vi "UHR-Fleezers Control (host) -Leonardo 04-2018 V3_greenctrl.vi"(0 "Tab Green FB":T5(tab)=enum."Trap Control (RF)") -> ()   [LabVIEW 2013] (continued)
              }
              n1852 = for {
                tunnel: w3550 -> [w3569] mode=indexing
                tunnel: [w3568] -> w3560 mode=indexing
                workers-P: _ -> [_]
                n1853 = Unbundle By Name(w3569) -> ("magnitude"=w3568:dbl[])
              }
              n1854 = Transpose 2D Array(2D array=w3560) -> (transposed array=w3559:dbl[][])
              n1855 = for {
                tunnel: w3559 -> [w3567] mode=indexing
                tunnel: [w3566] -> w3558 mode=indexing
                workers-P: _ -> [_]
                n1856 = Add Array Elements(numeric array=w3567) -> (sum=w3566:dbl)
              }
              n1857 = Select(t=w3553, s=w3554, f=w3552) -> (s? t:f=w3551:dbl)
              n1858 = Divide(x=w3558, y=w3551) -> (x/y=w3556:dbl[])
              n1859 = Bundle By Name(cluster=w3557, "magnitude"=w3556) -> (w3555:cluster{"f0":dbl, "df":dbl, "magnitude":dbl[]})
            }
          }
        }
        n1860 = case shown="True" w3497 {
          tunnel: w3498 -> [w3529 w3535]
          tunnel: [w3529 w3530] -> w3496
          frame False {
          }
          frame True {
            n1861 = Array Subset(array=w3535, index (row)=0 ("index"), length (row)=4 ("length"), index (col)=0 ("index"), length (col)=1 ("length")) -> (w3530:T47)
          }
        }
        n1862 = feedback-in #9(w3496) -> ()
        n1863 = Split 1D Array(array=w3510, index=2) -> (first subarray=→"FFT 1":cluster{"f0":dbl, "df":dbl, "magnitude":dbl[]}[], second subarray=→"FFT 2":cluster{"f0":dbl, "df":dbl, "magnitude":dbl[]}[])
      }
    }
    n1864 = Index Array(array=w2392, index=1) -> (element=w2400:waveform(dbl))
    n1865 = case "For displaying the high resolution display (no downsampling)" shown="True" w2456 {
      tunnel: w2419 -> [_ w2738]
      frame False {
      }
      frame True {
        n1866 = Index Array(array=w2738, index="High Res. Display") -> (element=w2739:waveform(dbl))
        n1867 = call <vilib>:"Std Deviation and Variance.vi"("X"=w2739) -> ("mean"=w2746:dbl, "standard deviation"=w2751:dbl)  [unwired: 1 in, 1 out]
        "Mean Intensity" <- w2746
        "Sigma" <- w2751
        n1868 = Subtract(x=w2739, y=w2746) -> (x-y=w2745:waveform(dbl))
        n1869 = Select(t=w2745, s="Subtract mean", f=w2739) -> (s? t:f=→"1 Channel":waveform(dbl))
        n1870 = Divide(x=w2751, y=w2746) -> (x/y=→"Sigma/Mean":dbl)
        n1871 = feedback #10(1) -> (w2740:i32)
        n1872 = Greater Or Equal?(x=w2740, y="Slow mean N ave.") -> (x >= y?=w2753:bool)
        n1873 = Increment(x=w2740) -> (x+1=w2755:i32)
        n1874 = Select(t=1, s=w2753, f=w2755) -> (s? t:f=w2742:i32)
        n1875 = feedback-in #10(w2742) -> ()
        n1876 = feedback #11() -> (w2743:waveform(dbl))  [unwired: 1 out]
        n1877 = case shown="Default" w2740 {
          tunnel: [w2758 w2761] -> w2744
          tunnel: w2743 -> [w2760 _]
          tunnel: w2739 -> [w2759 w2761]
          frame Default {
            n1878 = call-poly <vilib>:"Append Waveforms.vi"("waveform B"=w2759, "waveform A"=w2760) -> ("waveform out"=w2758:waveform(dbl))  [unwired: 1 in, 8 out]
          }
          frame 1 {
          }
        }
        n1879 = feedback-in #11(w2744) -> ()
        n1880 = case shown="True" w2753 {
          tunnel: w2744 -> [_ w2757]
          frame False {
          }
          frame True {
            n1881 = call-poly <vilib>:"Mean.vi"("X"=w2757) -> ("mean"=→"Slow mean":dbl)  [unwired: 1 out]
          }
        }
      }
    }
    n1882 = case "For plotting results of scanning MCL" shown="True" w2526 {
      tunnel: w2525 -> [_ w2878]
      tunnel: w2449 -> [_ w2974]
      tunnel: w2534 -> [_ _]
      tunnel: w2419 -> [_ w2948]
      tunnel: w2394 -> [_ w2879]
      tunnel: w2393 -> [_ w2852]
      frame False {
      }
      frame True {
        w2859 = u32 0 items=["Horizontal", "Vertical", "Central", "1st Diagonal", "2nd Diagonal"] ("Type of Symmetry")
        w2887 = u32 0 items=["Horizontal", "Vertical", "Central", "1st Diagonal", "2nd Diagonal"] ("Type of Symmetry")
        w2890 = u32 0 items=["Horizontal", "Vertical", "Central", "1st Diagonal", "2nd Diagonal"] ("Type of Symmetry")
        w2919 = u32 0 items=["Horizontal", "Vertical", "Central", "1st Diagonal", "2nd Diagonal"] ("Type of Symmetry")
        n1883 = Index Array(array=w2948, index=10) -> (element=w2954:waveform(dbl))
        n1884 = Index Array(array=w2948, index=11) -> (element=w2951:waveform(dbl))
        n1885 = local read "Cycles/step (MCL)"() -> (w2904:u64)
        n1886 = Index Array(array=w2948, index="Channel") -> (element=w2950:waveform(dbl))
        n1887 = Unbundle(w2852) -> ("New Image"=w2851:T3, "New Image"=w2850:T3, "New Image"=w2849:T3, "New Image"=w2848:T3)
        n1888 = Unbundle By Name(w2954) -> ("Y"=w2906:dbl[])
        n1889 = Unbundle By Name(w2951) -> ("Y"=w2908:dbl[])
        n1890 = Unbundle By Name(w2950) -> ("Y"=w2913:dbl[])
        n1891 = call "downsample 1D array - double.vi"("Ave N"=w2904, "Array In"=w2906) -> ("Array Out"=w2905:dbl[])  [unwired: 1 out]
        n1892 = call "downsample 1D array - double.vi"("Ave N"=w2904, "Array In"=w2908) -> ("Array Out"=w2907:dbl[])  [unwired: 1 out]
        n1893 = call "downsample 1D array - double.vi"("Ave N"=w2904, "Array In"=w2913) -> ("Array Out"=w2912:dbl[])  [unwired: 1 out]
        n1894 = feedback #12(w2974) -> (w2975:dbl[])
        n1895 = Build Array (concatenate)(w2975, w2974) -> (w2956:dbl[])
        n1896 = feedback #13(w2879) -> (w2881:dbl[])
        n1897 = Build Array (concatenate)(w2881, w2879) -> (w2880:dbl[])
        n1898 = local read "Scan steps (MCL)"() -> (w2861:u64)
        n1899 = Select(t=w2974, s=w2878, f=w2956) -> (s? t:f=w2960:dbl[])
        n1900 = feedback-in #12(w2960) -> ()
        n1901 = Select(t=w2879, s=w2878, f=w2880) -> (s? t:f=w2862:dbl[])
        n1902 = feedback-in #13(w2862) -> ()
        n1903 = local read "Scan lines (y)"() -> (w2847:u64)
        n1904 = local read "N APD Samp/step"() -> (w2863:dbl)
        n1905 = feedback #14(w2905) -> (w2962:dbl[])
        n1906 = Build Array (concatenate)(w2962, w2905) -> (w2953:dbl[])
        n1907 = feedback #15(w2912) -> (w2972:dbl[])
        n1908 = Build Array (concatenate)(w2972, w2912) -> (w2971:dbl[])
        n1909 = feedback #16(w2907) -> (w2964:dbl[])
        n1910 = Build Array (concatenate)(w2964, w2907) -> (w2965:dbl[])
        n1911 = Select(t=w2905, s=w2878, f=w2953) -> (s? t:f=w2909:dbl[])
        n1912 = feedback-in #14(w2909) -> ()
        n1913 = Select(t=w2912, s=w2878, f=w2971) -> (s? t:f=w2911:dbl[])
        n1914 = feedback-in #15(w2911) -> ()
        n1915 = Select(t=w2907, s=w2878, f=w2965) -> (s? t:f=w2910:dbl[])
        n1916 = feedback-in #16(w2910) -> ()
        n1917 = Multiply(x=w2861, y=u64 2) -> (x*y=w2846:u64)
        n1918 = call "integrate 1D array interval - double.vi"("Ave N"=w2863, "Array In"=w2862) -> ("Array Out"=w2874:dbl[])  [unwired: 1 out]
        n1919 = call "integrate 1D array interval - double.vi"("Ave N"=w2863, "Array In"=w2960) -> ("Array Out"=w2959:dbl[])  [unwired: 1 out]
        n1920 = Array Size(array=w2874) -> (size(s)=w2875:i32)
        n1921 = Array Size(array=w2959) -> (size(s)=w2961:i32)
        n1922 = Multiply(x=w2847, y=w2846) -> (x*y=w2877:u64)
        n1923 = Multiply(x=w2847, y=w2846) -> (x*y=w2969:u64)
        n1924 = call-poly <vilib>:"Mean.vi"("X"=w2909) -> ("mean"=w2893:dbl)  [unwired: 1 out]
        n1925 = Subtract(x=w2877, y=w2875) -> (x-y=w2868:u64)
        n1926 = call-poly <vilib>:"Mean.vi"("X"=w2911) -> ("mean"=w2898:dbl)  [unwired: 1 out]
        n1927 = call-poly <vilib>:"Mean.vi"("X"=w2910) -> ("mean"=w2896:dbl)  [unwired: 1 out]
        n1928 = call-poly <vilib>:"Mean.vi"("X"=w2874) -> ("mean"=w2865:dbl)  [unwired: 1 out]
        n1929 = Subtract(x=w2969, y=w2961) -> (x-y=w2903:u64)
        n1930 = call-poly <vilib>:"Mean.vi"("X"=w2959) -> ("mean"=w2900:dbl)  [unwired: 1 out]
        n1931 = Initialize Array(1.0 ("element"), w2868) -> (w2864:dbl[])
        n1932 = Initialize Array(1.0 ("element"), w2903) -> (w2894:dbl[])
        n1933 = Multiply(x=w2864, y=w2865) -> (x*y=w2866:dbl[])
        n1934 = Multiply(x=w2894, y=w2896) -> (x*y=w2897:dbl[])
        n1935 = Multiply(x=w2894, y=w2898) -> (x*y=w2899:dbl[])
        n1936 = Multiply(x=w2894, y=w2893) -> (x*y=w2895:dbl[])
        n1937 = Multiply(x=w2894, y=w2900) -> (x*y=w2901:dbl[])
        n1938 = Build Array (concatenate)(w2909, w2895) -> (w2963:dbl[])
        n1939 = Build Array (concatenate)(w2911, w2899) -> (w2967:dbl[])
        n1940 = Build Array (concatenate)(w2910, w2897) -> (w2966:dbl[])
        n1941 = Build Array (concatenate)(w2874, w2866) -> (w2876:dbl[])
        n1942 = Build Array (concatenate)(w2959, w2901) -> (w2968:dbl[])
        n1943 = Reshape Array(w2963, w2847, w2846) -> (w2929:dbl[][])
        n1944 = Reshape Array(w2876, w2847, w2846) -> (w2872:dbl[][])
        n1945 = Reshape Array(w2967, w2847, w2846) -> (w2921:dbl[][])
        n1946 = Reshape Array(w2966, w2847, w2846) -> (w2936:dbl[][])
        n1947 = Reshape Array(w2968, w2847, w2846) -> (w2946:dbl[][])
        n1948 = Array Subset(array=w2936, index (col)=0 ("index"), length (col)=w2861) -> (w2941:dbl[][])  [unwired: 2 in]
        n1949 = Array Subset(array=w2936, index (col)=w2861) -> (w2939:dbl[][])  [unwired: 3 in]
        n1950 = Array Subset(array=w2921, index (col)=0 ("index"), length (col)=w2861) -> (w2927:dbl[][])  [unwired: 2 in]
        n1951 = Array Subset(array=w2921, index (col)=w2861) -> (w2925:dbl[][])  [unwired: 3 in]
        n1952 = Array Subset(array=w2872, index (col)=0 ("index"), length (col)=w2861) -> (w2871:dbl[][])  [unwired: 2 in]
        n1953 = Array Subset(array=w2872, index (col)=w2861) -> (w2869:dbl[][])  [unwired: 3 in]
        n1954 = Array Subset(array=w2946, index (col)=0 ("index"), length (col)=w2861) -> (w2945:dbl[][])  [unwired: 2 in]
        n1955 = Array Subset(array=w2946, index (col)=w2861) -> (w2943:dbl[][])  [unwired: 3 in]
        n1956 = Array Subset(array=w2929, index (col)=0 ("index"), length (col)=w2861) -> (w2934:dbl[][])  [unwired: 2 in]
        n1957 = Array Subset(array=w2929, index (col)=w2861) -> (w2932:dbl[][])  [unwired: 3 in]
        n1958 = for {
          tunnel: w2941 -> [w2983] mode=indexing
          tunnel: [w2982] -> w2940 mode=indexing
          workers-P: _ -> [_]
          n1959 = Reverse 1D Array(array=w2983) -> (reversed array=w2982:dbl[])
        }
        n1960 = for {
          tunnel: w2927 -> [w2979] mode=indexing
          tunnel: [w2978] -> w2926 mode=indexing
          workers-P: _ -> [_]
          n1961 = Reverse 1D Array(array=w2979) -> (reversed array=w2978:dbl[])
        }
        n1962 = for {
          tunnel: w2871 -> [w2977] mode=indexing
          tunnel: [w2976] -> w2870 mode=indexing
          workers-P: _ -> [_]
          n1963 = Reverse 1D Array(array=w2977) -> (reversed array=w2976:dbl[])
        }
        n1964 = for {
          tunnel: w2945 -> [w2985] mode=indexing
          tunnel: [w2984] -> w2944 mode=indexing
          workers-P: _ -> [_]
          n1965 = Reverse 1D Array(array=w2985) -> (reversed array=w2984:dbl[])
        }
        n1966 = for {
          tunnel: w2934 -> [w2981] mode=indexing
          tunnel: [w2980] -> w2933 mode=indexing
          workers-P: _ -> [_]
          n1967 = Reverse 1D Array(array=w2981) -> (reversed array=w2980:dbl[])
        }
        n1968 = Index Array(array=w2946, index (row)=0) -> (element=→"Waveform Graph":dbl[])  [unwired: 1 in]
        n1969 = Add(x=w2940, y=w2939) -> (x+y=w2938:dbl[][])
        n1970 = Add(x=w2926, y=w2925) -> (x+y=w2924:dbl[][])
        n1971 = Add(x=w2870, y=w2869) -> (x+y=w2854:dbl[][])
        n1972 = Add(x=w2944, y=w2943) -> (x+y=w2918:dbl[][])
        n1973 = Add(x=w2933, y=w2932) -> (x+y=w2931:dbl[][])
        n1974 = Divide(x=w2924, y=2) -> (x/y=w2922:dbl[][])
        n1975 = Divide(x=w2938, y=2) -> (x/y=w2883:dbl[][])
        n1976 = Divide(x=w2931, y=2) -> (x/y=w2885:dbl[][])
        n1977 = To Single Precision Float(number=w2918) -> (single precision float=w2917:sgl[][])
        n1978 = Transpose 2D Array(2D array=w2922) -> (transposed array=→"Data map":dbl[][])
        n1979 = To Single Precision Float(number=w2854) -> (single precision float=w2858:sgl[][])
        n1980 = To Single Precision Float(number=w2883) -> (single precision float=w2889:sgl[][])
        n1981 = To Single Precision Float(number=w2885) -> (single precision float=w2886:sgl[][])
        n1982 = call "IMAQ ArrayToImage"("Image Pixels (Float)"=w2917, "Image"=w2851) -> ("Image Out"=w2920:T3)  [unwired: 8 in, 1 out]
        n1983 = call "IMAQ ArrayToImage"("Image Pixels (Float)"=w2858, "Image"=w2850) -> ("Image Out"=w2860:T3)  [unwired: 8 in, 1 out]
        n1984 = call "IMAQ ArrayToImage"("Image Pixels (Float)"=w2889, "Image"=w2849) -> ("Image Out"=w2891:T3)  [unwired: 8 in, 1 out]
        n1985 = call "IMAQ ArrayToImage"("Image Pixels (Float)"=w2886, "Image"=w2848) -> ("Image Out"=w2888:T3)  [unwired: 8 in, 1 out]
        n1986 = call "IMAQ Symmetry"("Type of Symmetry"=w2919, "Image Src"=w2920) -> ("Image Dst Out"=w2915:T3)  [unwired: 3 in, 1 out]
        n1987 = call "IMAQ Symmetry"("Type of Symmetry"=w2859, "Image Src"=w2860) -> ("Image Dst Out"=w2856:T3)  [unwired: 3 in, 1 out]
        n1988 = call "IMAQ Symmetry"("Type of Symmetry"=w2890, "Image Src"=w2891) -> ("Image Dst Out"=→"Detection Laser X":T3)  [unwired: 3 in, 1 out]
        n1989 = call "IMAQ Symmetry"("Type of Symmetry"=w2887, "Image Src"=w2888) -> ("Image Dst Out"=→"Detection Laser Y":T3)  [unwired: 3 in, 1 out]
        n1990 = call "IMAQ Set Simple Calibration"("Calibration Axis Info"=T37 {"Origin Pixel"={"X"=0.0, "Y"=0.0}, "Angle Relative to Horizontal (deg)"=0.0, "Axis Reference"=0}, "Grid Descriptor"=T38 {"X Step"=0.3, "Y Step"=0.3, "Unit"=enum."Undefined"}, "Image"=w2915) -> ("Calibrated Image"=→"APD 1":T3)  [unwired: 7 in, 1 out]
        n1991 = call "IMAQ Set Simple Calibration"("Calibration Axis Info"=T37 {"Origin Pixel"={"X"=0.0, "Y"=0.0}, "Angle Relative to Horizontal (deg)"=0.0, "Axis Reference"=0}, "Grid Descriptor"=T38 {"X Step"=0.3, "Y Step"=0.3, "Unit"=enum."Undefined"}, "Image"=w2856) -> ("Calibrated Image"=→"APD 2":T3)  [unwired: 7 in, 1 out]
      }
    }
    n1992 = Subtract(x=w2400, y="APD 2 Offset") -> (x-y=w2397:waveform(dbl))
    n1993 = Subtract(x=w2402, y="APD 1 Offset") -> (x-y=w2398:waveform(dbl))
    n1994 = Index Array(array=w2417, index=3) -> (element=w2476:waveform(dbl))
    n1995 = Index Array(array=w2417, index=6) -> (element=w2473:waveform(dbl))
    n1996 = Build Array(w2398, w2397) -> (→"APD Chart":waveform(dbl)[])
    n1997 = Array Size(array=w2466) -> (size(s)=w2514:i32)
    n1998 = call <vilib>:"Std Deviation and Variance.vi"("X"=w2410) -> ("standard deviation"=w2409:dbl)  [unwired: 1 in, 2 out]
    n1999 = Add Array Elements(numeric array=w2410) -> (sum=w2412:u32)
    n2000 = Add Array Elements(numeric array=w2466) -> (sum=w2524:u32)
    n2001 = call <vilib>:"Std Deviation and Variance.vi"("X"=w2466) -> ("standard deviation"=w2465:dbl)  [unwired: 1 in, 2 out]
    n2002 = Divide(x=w2409, y=w2408) -> (x/y=w2405:dbl)
    "Rate sigma (Hz) 2" <- w2405
    n2003 = Multiply(x=w2408, y=w2514) -> (x*y=w2411:dbl)
    "Int. Time (s)" <- w2411
    n2004 = Divide(x=w2412, y=w2411) -> (x/y=w2406:dbl)
    "APD 2 Rate (Hz)" <- w2406
    n2005 = Divide(x=w2524, y=w2411) -> (x/y=w2463:dbl)
    "APD 1 Rate (Hz)" <- w2463
    n2006 = Divide(x=w2465, y=w2408) -> (x/y=w2464:dbl)
    "Rate sigma (Hz)" <- w2464
    n2007 = Divide(x=w2405, y=w2406) -> (x/y=→"Sigma/Mean 2":dbl)
    n2008 = Divide(x=w2464, y=w2463) -> (x/y=→"Sigma/Mean":dbl)
    n2009 = case shown="2" "Calibration" {
      tunnel: "T1 alpha_x (nm/V)" -> [_ w2814 w2835]
      tunnel: "T1 kappa_x (pN/nm)" -> [_ _ w2825]
      tunnel: "T2 alpha_x (nm/V)" -> [_ w2813 w2833]
      tunnel: "T2 kappa_x (pN/nm)" -> [_ _ w2826]
      tunnel: w2476 -> [w2796 w2811 w2831]
      tunnel: w2473 -> [w2795 w2809 w2829]
      tunnel: [w2796 w2808 w2828] -> w2266
      tunnel: [w2795 w2807 w2827] -> w2272
      tunnel: ["T1 X (V)" ("Label.Text") "T1 X (nm)" ("Label.Text") "T1 X (pN)" ("Label.Text")] -> w2494
      tunnel: ["T2 X (V)" ("Label.Text") "T2 X (nm)" ("Label.Text") "T2 X (pN)" ("Label.Text")] -> w2493
      tunnel: ["Position (V)" ("Label.Text") "Position (nm)" ("Label.Text") "Force (pN)" ("Label.Text")] -> w2495
      tunnel: w2475 -> [_ w2799 w2818]
      tunnel: w2477 -> [_ w2802 w2820]
      tunnel: ["Mean (V)" ("Label.Text") "Mean (nm)" ("Label.Text") "Mean (pN)" ("Label.Text")] -> w2490
      tunnel: ["Difference (V)" ("Label.Text") "Difference (nm)" ("Label.Text") "Difference (pN)" ("Label.Text")] -> w2425
      frame 0, Default {
      }
      frame 1 {
        # "position"
        n2010 = Unbundle By Name(w2811) -> ("Y"=w2815:dbl[])
        n2011 = Unbundle By Name(w2809) -> ("Y"=w2800:dbl[])
        n2012 = Subtract(x=w2815, y=w2802) -> (x-y=w2803:dbl[])
        n2013 = Subtract(x=w2800, y=w2799) -> (x-y=w2801:dbl[])
        n2014 = Multiply(x=w2801, y=w2813) -> (x*y=w2810:dbl[])
        n2015 = Multiply(x=w2814, y=w2803) -> (x*y=w2812:dbl[])
        n2016 = Bundle By Name(cluster=w2809, "Y"=w2810) -> (w2807:waveform(dbl))
        n2017 = Bundle By Name(cluster=w2811, "Y"=w2812) -> (w2808:waveform(dbl))
      }
      frame 2 {
        # "force"
        n2018 = Unbundle By Name(w2831) -> ("Y"=w2836:dbl[])
        n2019 = Unbundle By Name(w2829) -> ("Y"=w2834:dbl[])
        n2020 = Subtract(x=w2834, y=w2818) -> (x-y=w2819:dbl[])
        n2021 = Subtract(x=w2836, y=w2820) -> (x-y=w2821:dbl[])
        n2022 = Compound Arithmetic op=MULTIPLY(w2819, w2833, w2826) -> (w2830:dbl[])
        n2023 = Compound Arithmetic op=MULTIPLY(w2825, w2835, w2821) -> (w2832:dbl[])
        n2024 = Bundle By Name(cluster=w2829, "Y"=w2830) -> (w2827:waveform(dbl))
        n2025 = Bundle By Name(cluster=w2831, "Y"=w2832) -> (w2828:waveform(dbl))
      }
    }
    n2026 = feedback-in #17("Calibration") -> ()
    n2027 = feedback #17(u16 1 ("Calibration")) -> (w2497:u16)
    n2028 = local read "Trap 2 Bead Size (nm)"() -> (w2305:dbl)
    n2029 = local read "Trap 1 Bead Size (nm)"() -> (w2304:dbl)
    n2030 = local read "AOM X Cal (nm/MHz)"() -> (w2302:dbl)
    n2031 = local read "Trap Delta (MHz)"() -> (w2301:dbl)
    n2032 = Not Equal?(x=w2497, y="Calibration") -> (x != y?=w2454:bool)
    n2033 = Multiply(x=w2302, y=w2301) -> (x*y=w2306:dbl)
    n2034 = Unbundle By Name(w2266) -> ("Y"=w2271:dbl[])
    n2035 = Unbundle By Name(w2272) -> ("Y"=w2270:dbl[])
    n2036 = Add(x=w2305, y=w2304) -> (x+y=w2308:dbl)
    n2037 = case shown="False" "Negate trap 2 force" {
      tunnel: [-1.0 1.0] -> w2483
      frame False {
      }
      frame True {
      }
    }
    n2038 = Unbundle By Name(w2476) -> ("Y"=w2479:dbl[])
    n2039 = Unbundle By Name(w2473) -> ("Y"=w2482:dbl[])
    n2040 = Divide(x=w2308, y=2.0) -> (x/y=w2303:dbl)
    n2041 = Subtract(x=w2271, y=w2270) -> (x-y=w2268:dbl[])
    n2042 = Subtract(x=w2479, y=w2477) -> (x-y=w2480:dbl[])
    n2043 = Subtract(x=w2482, y=w2475) -> (x-y=w2481:dbl[])
    n2044 = Divide(x=w2268, y=2.0) -> (x/y=w2267:dbl[])
    n2045 = Multiply(x=w2481, y="T2 alpha_x (nm/V)") -> (x*y=w2472:dbl[])
    n2046 = Multiply(x="T1 alpha_x (nm/V)", y=w2480) -> (x*y=w2471:dbl[])
    n2047 = Multiply(x=w2272, y=w2483) -> (x*y=w2484:waveform(dbl))
    n2048 = Bundle By Name(cluster=w2266, "Y"=w2267) -> (w2265:waveform(dbl))
    n2049 = case shown="True" "Read Lateness and Rel Phase" {
      tunnel: w2278 -> [w2762 w2784]
      tunnel: w2317 -> [w2763 w2783]
      tunnel: [w2762 w2782] -> w2469
      tunnel: [w2763 w2781] -> w2468
      frame False {
      }
      frame True {
        n2050 = xnode "Read/Write Control"("FPGA VI Reference In"=w2784, "error in"=w2783) -> ("FPGA VI Reference Out"=w2782:T20, "error out"=w2781:errorcluster, "GI Relative phase"=→"GI relative phase":i16, "Relative phase"=→"Relative phase (AI1)":i16, "AI Late Counter"=→"Late Counter (AI1)":u8, "GI Late Counter"=→"GI Late Counter":u8, "MCL Late Counter"=→"MCL Late Counter":u8, "MCL Relative Phase"=→"Relative Phase (MCL)":i16, "APD Acq Relative Phase"=→"APD Acq Relative Phase":i16, "APD 1 Gate Relative Phase"=→"APD 1 Gate Relative Phase":i16, "APD 2 Gate Relative Phase"=→"APD 2 Gate Relative Phase":i16, "APD Acq Late Counter"=→"APD Acq Late Counter":u16, "APD 1 Gate Late Counter"=→"APD 1 Gate Late Counter":u8, "APD 2 Gate Late Counter"=→"APD 2 Gate Late Counter":u8, "Green FB Relative Phase"=→"Relative phase (Green FB)":i16, "GI Relative phase"=→"GI relative phase 2":i16, "GI Late Counter 2"=→"GI Late Counter 2":u16, "Trap Pos FIFO Timeout"=→"Trap Pos FIFO Timeout":u16, "Trap AI FIFO Timeout"=→"Trap AI FIFO Timeout":u16)
      }
    }
    n2051 = Subtract(x=w2472, y=w2471) -> (x-y=w2300:dbl[])
    n2052 = call-poly <vilib>:"Mean.vi"("X"=w2300) -> ("mean"=w2307:dbl)  [unwired: 1 out]
    n2053 = Add(x=w2306, y=w2307) -> (x+y=w2310:dbl)
    n2054 = Subtract(x=w2310, y=w2303) -> (x-y=→"Tether Extension (nm, calculated)":dbl)
    n2055 = Unbundle By Name(w2272) -> ("Y"=w2263:dbl[])
    n2056 = Unbundle By Name(w2266) -> ("Y"=w2264:dbl[])
    n2057 = Build Array(w2266, w2484, w2265) -> (→"Force":waveform(dbl)[])
    n2058 = Subtract(x=w2300, y="Offset (nm)") -> (x-y=w2444:dbl[])
    n2059 = call-poly <vilib>:"Mean.vi"("X"=w2263) -> ("mean"=w2261:dbl)  [unwired: 1 out]
    "T2 X" <- w2261
    n2060 = call-poly <vilib>:"Mean.vi"("X"=w2264) -> ("mean"=w2262:dbl)  [unwired: 1 out]
    "T1 X" <- w2262
    n2061 = Subtract(x=w2264, y=w2263) -> (x-y=w2446:dbl[])
    n2062 = Bundle By Name(cluster=w2476, "Y"=w2444) -> (w2416:waveform(dbl))
    "Bead Separation" <- w2416
    n2063 = Divide(x=w2446, y=2.0) -> (x/y=→"Vec Mean of T1 T2":dbl[])
    n2064 = case shown="True" w2454 {
      tunnel: w2495 -> [_ w2789]
      tunnel: w2494 -> [_ w2788]
      tunnel: w2493 -> [_ w2787]
      tunnel: w2490 -> [_ w2786]
      tunnel: w2425 -> [_ w2785]
      frame False {
      }
      frame True {
        n2065 = property on="Force" class="WFChart (strict)"("YScale.NameLbl.Text"=w2789) -> ()  [unwired: 2 in, 2 out]
        n2066 = property on="T2 X" class="DigNum (strict)"("Caption.Text"=w2787) -> ()  [unwired: 2 in, 2 out]
        n2067 = property on="T1 X" class="DigNum (strict)"("Caption.Text"=w2788) -> ()  [unwired: 2 in, 2 out]
        n2068 = property on="Mean" class="DigNum (strict)"("Caption.Text"=w2786) -> ()  [unwired: 2 in, 2 out]
        n2069 = property on="Difference" class="DigNum (strict)"("Caption.Text"=w2785) -> ()  [unwired: 2 in, 2 out]
      }
    }
    n2070 = local read "Tether"() -> (w2448:bool)
    n2071 = Subtract(x=w2262, y=w2261) -> (x-y=w2492:dbl)
    n2072 = Add(x=w2262, y=w2261) -> (x+y=→"Difference":dbl)
    n2073 = feedback #18(w2444) -> (w2443:dbl[])
    n2074 = Divide(x=w2492, y=2.0) -> (x/y=w2275:dbl)
    "Mean" <- w2275
    n2075 = case shown="True" w2448 {
      tunnel: w2275 -> [_ w2721]
      frame False {
      }
      frame True {
        n2076 = Greater?(x="Lost Tether Alarm Threshold (pN)", y=w2721) -> (0:w2719:bool)
        n2077 = case shown="True" w2719 {
          frame False {
          }
          frame True {
            n2078 = flat-sequence {
              frame #0 {
                # "stop only if saving"
                n2079 = local read "Saving..."() -> (w2734:bool)
                n2080 = And(x=w2734, y="TA Cancel Save?") -> (x .and. y?=w2733:bool)
                n2081 = local write "Stop Saving"(w2733) -> ()
              }
              frame #1 {
                n2082 = case shown="True" "TA Green Off?" {
                  frame False {
                  }
                  frame True {
                    w2737 = FALSE ("Fl. Triggered...")
                    n2083 = local write "Fl. Triggered..."(w2737) -> ()
                    n2084 = property on="Green Laser ON/Interlacing" class="Bool (strict)"("Val(Sgnl)"=w2737) -> ()  [unwired: 2 in, 2 out]
                  }
                }
              }
            }
            n2085 = local read "Time tether formed"() -> (w2728:timestamp)
            n2086 = Get Date/Time In Seconds() -> (seconds since 1Jan1904=w2729:timestamp)
            n2087 = Subtract(x=w2729, y=w2728) -> (x-y=w2727:dbl)
            n2088 = Number To Decimal String(number=w2727) -> (decimal integer string=w2724:string)  [unwired: 1 out]
            n2089 = local read "Messages"() -> (w2731:string)
            n2090 = call <vilib>:"Beep.vi"() -> ()  [unwired: 3 in, 9 out]
            n2091 = Concatenate Strings("Lost tether (" ("Message to add"), w2724, " s)." ("string")) -> (w2726:string)
            n2092 = local write "Tether"(FALSE ("Tether")) -> ()
            n2093 = call "Update messages.vi"("Message to add"=w2726, "Old message string"=w2731) -> ("New message string"=w2730:string)
            n2094 = local write "Messages"(w2730) -> ()
            n2095 = property on="Trap Pos. FB ON" class="Bool (strict)"("Val(Sgnl)"=FALSE ("Value (Signaling)")) -> ()  [unwired: 2 in, 2 out]
          }
        }
      }
    }
    n2096 = Build Array (concatenate)(w2444, w2443) -> (w2442:dbl[])
    n2097 = Split 1D Array(array=w2442, index=w2328) -> (first subarray=w2438:dbl[])  [unwired: 1 out]
    n2098 = feedback-in #18(w2438) -> ()
    n2099 = call-poly <vilib>:"Mean.vi"("X"=w2438) -> ("mean"=w2437:dbl)  [unwired: 1 out]
    "Bead Mean (nm)" <- w2437
    n2100 = Subtract(x=w2438, y=w2437) -> (x-y=w2436:dbl[])
    n2101 = Square(x=w2436) -> (x^2=w2435:dbl[])
    n2102 = case shown="True" "Semi Passive ON" {
      tunnel: "Semi Passive mode" -> [_ w2602]
      tunnel: "Jump Force (pN)" -> [_ w2601]
      tunnel: w2275 -> [_ w2600]
      frame False {
      }
      frame True {
        n2103 = case shown="\"Use Feedback\"" w2602 {
          tunnel: w2601 -> [_ w2605 w2621]
          tunnel: w2600 -> [_ w2604 w2620]
          frame "None" {
          }
          frame "Use Feedback" {
            n2104 = local read "Target Force (pN)"() -> (w2607:dbl)
            n2105 = Less?(x=w2605, y=w2607) -> (x < y?=w2606:bool)
            n2106 = case shown="True" w2606 {
              tunnel: w2605 -> [w2614 w2617]
              tunnel: w2604 -> [w2613 w2616]
              tunnel: [w2612 w2615] -> w2603
              frame False {
                n2107 = Less?(x=w2614, y=w2613) -> (x < y?=w2612:bool)
              }
              frame True {
                n2108 = Greater?(x=w2617, y=w2616) -> (0:w2615:bool)
              }
            }
            n2109 = case shown="True" w2603 {
              frame False {
                n2110 = local read "Trap Pos. FB ON"() -> (w2608:bool)
                n2111 = case shown="True" w2608 {
                  frame False {
                  }
                  frame True {
                    n2112 = property on="Trap Pos. FB ON" class="Bool (strict)"("Val(Sgnl)"=FALSE) -> ()  [unwired: 2 in, 2 out]
                  }
                }
              }
              frame True {
                n2113 = local read "Trap Pos. FB ON"() -> (w2610:bool)
                n2114 = case shown="False" w2610 {
                  frame False {
                    n2115 = property on="Trap Pos. FB ON" class="Bool (strict)"("Val(Sgnl)"=TRUE) -> ()  [unwired: 2 in, 2 out]
                  }
                  frame True {
                  }
                }
              }
            }
          }
          frame "Sharp Jump" {
            n2116 = local read "Target Force (pN)"() -> (w2623:dbl)
            n2117 = Greater?(x=w2621, y=w2623) -> (0:w2622:bool)
            n2118 = case shown="True" w2622 {
              tunnel: w2621 -> [w2638 w2642]
              tunnel: w2620 -> [w2639 w2641]
              tunnel: [w2637 w2640] -> w2619
              frame False {
                n2119 = Greater?(x=w2639, y=w2638) -> (0:w2637:bool)
              }
              frame True {
                n2120 = Less?(x=w2642, y=w2641) -> (x < y?=w2640:bool)
              }
            }
            n2121 = Subtract(x=w2621, y=w2623) -> (x-y=w2618:dbl)
            n2122 = case shown="True" w2619 {
              tunnel: w2618 -> [_ w2629]
              frame False {
              }
              frame True {
                n2123 = local read "T1 kappa_x (pN/nm)"() -> (w2634:dbl)
                n2124 = local read "T2 kappa_x (pN/nm)"() -> (w2635:dbl)
                n2125 = Reciprocal(x="DNA stiffness (pN / nm)") -> (1/x=w2631:dbl)
                n2126 = Reciprocal(x=w2634) -> (1/x=w2633:dbl)
                n2127 = Reciprocal(x=w2635) -> (1/x=w2632:dbl)
                n2128 = Compound Arithmetic op=ADD(w2633, w2632, w2631) -> (w2630:dbl)
                n2129 = local read "AOM X Cal (nm/MHz)"() -> (w2628:dbl)
                n2130 = Multiply(x=w2630, y=w2629) -> (x*y=w2627:dbl)
                n2131 = local read "Trap Delta (MHz)"() -> (w2625:dbl)
                n2132 = Divide(x=w2627, y=w2628) -> (x/y=w2626:dbl)
                n2133 = Subtract(x=w2625, y=w2626) -> (x-y=w2624:dbl)
                n2134 = property on="Trap Delta (MHz)" class="DigNum (strict)"("Val(Sgnl)"=w2624) -> ()  [unwired: 2 in, 2 out]
              }
            }
          }
        }
      }
    }
    n2135 = call-poly <vilib>:"Mean.vi"("X"=w2435) -> ("mean"=w2434:dbl)  [unwired: 1 out]
    n2136 = Square Root(x=w2434) -> (sqrt(x)=w2433:dbl)
    n2137 = Multiply(x=10.0, y=w2433) -> (x*y=→"RMS (Ang)":dbl)
    n2138 = xnode "Read/Write Control"("FPGA VI Reference In"=w2469, "error in"=w2468) -> ("FPGA VI Reference Out"=w2578:T20, "error out"=w2572:errorcluster, "AI2 Y Sum Set 1"=w2568:i16, "AI2 Y Sum Set 2"=w2567:i16, "AI1 X Set 1"=w2362:fxp<+/-,16,1>, "AI1 X Set 2"=w2361:fxp<+/-,16,1>, "Trap Pos FB Int Signal"=→"Trap Pos FB Int Signal":fxp<+/-,24,9>, "Trap Pos FB Int-Norm Signal"=→"Trap Pos FB Int-Norm Signal":fxp<+/-,16,1>, "Trap Pos FB Action"=w2355:i64, "Scanning"=→"AOD Scanning":bool, "Scan I"=→"AOD Scan I":u64, "Scanning MCL"=w2570:bool, "Scan I (MCL)"=→"MCL Scan I":u64, "Green FB Signals"=w2509:T48, "BD1 amplitude 1 out"=w2260:u16, "BD1 amplitude 2 out"=w2245:u16)  [unwired: 1 out]
    "MCL Scanning" <- w2570
    "Trap Pos FB Action" <- w2355
    n2139 = local read "AI2 (V)"() -> (w2569:cluster{"Set 1":dbl, "Set 2":dbl})
    n2140 = Bundle By Name(cluster=w2569, "Set 1"=w2568, "Set 2"=w2567) -> (w2565:cluster{"Set 1":dbl, "Set 2":dbl})
    n2141 = Divide(x=w2355, y=327.67) -> (x/y=→"Action (%)":dbl)
    n2142 = local read "Trap X (AI1)"() -> (w2375:T1)
    n2143 = Divide(x=w2565, y=3276.7) -> (x/y=w2564:cluster{"Set 1":dbl, "Set 2":dbl})
    n2144 = local write "AI2 (V)"(w2564) -> ()
    n2145 = Bundle(cluster=w2375, "Trap 1"=w2362, "Trap 2"=w2361) -> (→"Trap X (AI1)":T1)
    n2146 = Scale By Power Of 2(n=i16 12, x=ext 1.0) -> (x*2^n=w2256:ext)
    n2147 = Subtract(x=w2256, y=ext 1.0) -> (x-y=w2253:ext)
    n2148 = Divide(x=w2509, y=3276.7) -> (x/y=w2505:T49)
    n2149 = Multiply(x=w2260, y=ext 100.0) -> (x*y=w2254:ext)
    n2150 = Unbundle By Name(w2505) -> ("Green FB Ch 0"=w2508:dbl, "Green FB Ch 1"=w2507:dbl, "Green FB Ch 2"=w2506:dbl)
    n2151 = local read "All FB On/Off"() -> (w2244:bool)
    n2152 = Divide(x=w2254, y=w2253) -> (x/y=w2243:ext)
    "Trap 1 amplitude" <- w2243
    n2153 = Scale By Power Of 2(n=i16 12, x=ext 1.0) -> (x*2^n=w2249:ext)
    n2154 = Subtract(x=w2249, y=ext 1.0) -> (x-y=w2252:ext)
    n2155 = Multiply(x=w2245, y=ext 100.0) -> (x*y=w2251:ext)
    n2156 = Divide(x=w2508, y=w2506) -> (x/y=w2504:dbl)
    n2157 = Divide(x=w2507, y=w2506) -> (x/y=w2503:dbl)
    n2158 = flat-sequence "To save data" {
      tunnel: [w3618] -> w2589
      tunnel: [w3619] -> w2588
      tunnel: w2540 -> [w3612]
      tunnel: w2440 -> [w3616]
      tunnel: ["Save Calibration"] -> w2561
      tunnel: w2558 -> [w3615]
      tunnel: [w3608] -> w2557
      tunnel: [w3605] -> w2556
      tunnel: [w3602] -> w2555
      tunnel: w2539 -> [w3604]
      tunnel: w2452 -> [w3598]
      tunnel: [w3598] -> w2451
      tunnel: ["Start Saving"] -> w2418
      tunnel: [w3592] -> w2344
      tunnel: [w3591] -> w2343
      tunnel: w2589 -> [w3853]
      tunnel: w2588 -> [w3852]
      tunnel: w2345 -> [w3851]
      tunnel: w2561 -> [w3850]
      tunnel: w2557 -> [w3848]
      tunnel: w2556 -> [w3847]
      tunnel: w2555 -> [w3846]
      tunnel: w2427 -> [w3845]
      tunnel: w2461 -> [w3844]
      tunnel: w2451 -> [w3843]
      tunnel: w2418 -> [w3842]
      tunnel: w2416 -> [w3841]
      tunnel: w2392 -> [w3840]
      tunnel: w2344 -> [w3839]
      tunnel: w2343 -> [w3838]
      tunnel: w2342 -> [w3837]
      frame #0 {
        n2159 = Or(x="Save N Sets", y="Start Saving") -> (x .or. y?=w3599:bool)
        n2160 = To Double Precision Float(number=w3615) -> (double precision float=w3609:dbl)
        n2161 = Build Array(w3599, "Save Calibration", w3612, w3604) -> (w3614:bool[])
        n2162 = Compound Arithmetic op=OR("Save Calibration", w3612, w3599, w3604) -> (w3617:bool)
        n2163 = Boolean Array To Number(Boolean array=w3614) -> (number=w3611:u32)
        n2164 = feedback #19(FALSE ("Save APD Data\nwith Trap Data")) -> (w3593:bool)
        n2165 = feedback #20(refnum<k0> refnum) -> (w3620:refnum<file>)
        n2166 = feedback #21(refnum<k0> refnum) -> (w3595:refnum<file>)
        n2167 = feedback #22(FALSE ("Save APD Data\nwith Trap Data")) -> (w3603:bool)
        n2168 = feedback #23(refnum<k0> refnum) -> (w3606:refnum<file>)
        n2169 = feedback #24(0) -> (w3622:i32)
        n2170 = feedback #25() -> (w3610:u32)  [unwired: 1 out]
        n2171 = case shown="True" w3617 {
          tunnel: [w3629 1] -> w3618
          tunnel: w3622 -> [w3631 _]
          tunnel: [w3630 w3649] -> w3619
          tunnel: w3620 -> [w3630 _]
          tunnel: w3616 -> [_ w3669]
          tunnel: w3609 -> [_ w3667]
          tunnel: w3611 -> [_ w3670]
          tunnel: [w3628 w3648] -> w3608
          tunnel: w3610 -> [w3628 _]
          tunnel: [w3627 w3646] -> w3605
          tunnel: w3606 -> [w3627 _]
          tunnel: [w3626 w3645] -> w3602
          tunnel: w3603 -> [w3626 _]
          tunnel: "Start Saving" -> [_ w3643]
          tunnel: w3598 -> [_ w3642]
          tunnel: [w3625 w3633] -> w3591
          tunnel: w3595 -> [w3625 _]
          tunnel: [w3624 w3632] -> w3592
          tunnel: w3593 -> [w3624 _]
          frame False {
            n2172 = Increment(x=w3631) -> (x+1=w3629:i32)
          }
          frame True {
            w3639 = FALSE ("Start Saving")
            w3644 = 9.0  # File Version
            w3652 = FALSE ("prepend array or string size? (T)")
            w3650 = T30."big-endian, network order" ("byte order (0:big-endian, network order)")
            # "write file headers"
            n2173 = local read "BD 1 Frequency 1 (MHz)"() -> (w3666:dbl)
            n2174 = local read "BD 2 Frequency 1 (MHz)"() -> (w3665:dbl)
            n2175 = local read "BD 1 Frequency 2 (MHz)"() -> (w3664:dbl)
            n2176 = local read "BD 2 Frequency 2 (MHz)"() -> (w3663:dbl)
            n2177 = local read "BD 1 Frequency 3 (MHz)"() -> (w3662:dbl)
            n2178 = local read "BD 2 Frequency 3 (MHz)"() -> (w3661:dbl)
            n2179 = Array Size(array=w3642) -> (size(s)=w3641:i32)
            n2180 = To Double Precision Float(number=w3641) -> (double precision float=w3640:dbl)
            n2181 = local write "Save Calibration"(w3639) -> ()
            n2182 = local write "Start Saving"(w3639) -> ()
            n2183 = Build Array("Save APD Data\nwith Trap Data", "Save Trap Pos. Data") -> (w3636:bool[])
            n2184 = Boolean Array To Number(Boolean array=w3636) -> (number=w3635:u32)
            n2185 = Build Array(w3666, w3665, w3664, w3663, w3662, w3661) -> (w3660:dbl[])
            n2186 = case shown="2" w3670 {
              tunnel: w3669 -> [w3741 w3761 w3777 w3815]
              tunnel: w3640 -> [w3746 w3768 w3797 w3834]
              tunnel: w3667 -> [w3745 w3767 w3796 w3833]
              tunnel: [w3742 w3763 w3788 w3825] -> w3658
              tunnel: [w3733 "Cal sets to save" w3778 w3816] -> w3648
              tunnel: w3660 -> [w3743 w3764 w3790 w3827]
              tunnel: "Save APD Data\nwith Trap Data" -> [w3740 _ w3774 w3813]
              tunnel: [w3740 w3755 w3774 w3813] -> w3645
              tunnel: w3644 -> [w3736 w3756 w3772 w3811]
              tunnel: w3643 -> [w3735 _ _ _]
              tunnel: [w3726 w3755 w3771 w3801] -> w3632
              tunnel: "Save Trap Pos. Data" -> [w3726 _ w3771 w3801]
              tunnel: w3635 -> [w3725 _ w3770 w3800]
              frame 1, Default {
                # "timeseries"
                n2187 = case shown="True" "Profile" {
                  tunnel: [w3749 w3752] -> w3730
                  tunnel: [w3749 w3751] -> w3729
                  tunnel: [w3749 w3750] -> w3728
                  tunnel: [w3749 w3754] -> w3727
                  frame False {
                    w3749 = 0.0 ("f")
                  }
                  frame True {
                    n2188 = local read "Current Position"() -> (w3753:dbl[])
                    n2189 = local read "Y change (mm)"() -> (w3754:dbl)
                    n2190 = call "subVI_explode3array.vi"("Array"=w3753) -> ("x"=w3752:dbl, "y"=w3751:dbl, "z"=w3750:dbl)  [unwired: 12 in]
                  }
                }
                n2191 = local read "Save ave N"() -> (w3748:dbl)
                n2192 = Multiply(x=w3748, y=w3741) -> (x*y=w3747:dbl)
                n2193 = To Double Precision Float(number=w3725) -> (double precision float=w3739:dbl)
                n2194 = Build Array(w3736, w3741, w3747, w3746, w3745, 0.0 ("f")) -> (w3744:dbl[])
                n2195 = Build Array(w3739, w3730, w3729, w3728, w3727) -> (w3737:dbl[])
                n2196 = Select(t=u32 4000000000, s=w3735, f="N sets to save") -> (s? t:f=w3733:u32)
                n2197 = Build Array (concatenate)(w3744, w3743, w3737) -> (w3742:dbl[])
              }
              frame 2 {
                w3758 = 0.0 ("f")
                w3755 = FALSE ("Save APD Data\nwith Trap Data")
                # "calibration"
                n2198 = Boolean To (0,1)(Boolean=w3755) -> (0, 1=w3760:i16)
                n2199 = To Double Precision Float(number=w3760) -> (double precision float=w3759:dbl)
                n2200 = Build Array(w3759, w3758, w3758, w3758, w3758) -> (w3757:dbl[])
                n2201 = Build Array(w3756, w3761, w3761, w3768, w3767, 1.0 ("t")) -> (w3765:dbl[])
                n2202 = Build Array (concatenate)(w3765, w3764, w3757) -> (w3763:dbl[])
                "Calibrating Trap..." <- TRUE ("Calibrating...")
              }
              frame 4 {
                w3775 = 0.0 ("f")
                # "write file header for a trap \nraster scan"
                # "scan dir (x/y = 0/1)"
                # "cycles/step"
                # "n scans (f/b)"
                # "steps"
                # "freq. range"
                # "AOD raster scan"
                n2203 = local read "Number of F/B Scans (AOD)"() -> (w3782:u16)
                n2204 = local read "Cycles/step (AOD)"() -> (w3784:u64)
                n2205 = local read "Scan Range (MHz)"() -> (w3787:dbl)
                n2206 = local read "Scan steps (AOD)"() -> (w3786:u64)
                n2207 = local read "Scan BD"() -> (w3794:bool)
                n2208 = local read "Save ave N"() -> (w3799:dbl)
                n2209 = Boolean To (0,1)(Boolean=w3794) -> (0, 1=w3793:i16)
                n2210 = To Double Precision Float(number=w3782) -> (double precision float=w3781:dbl)
                n2211 = To Double Precision Float(number=w3786) -> (double precision float=w3785:dbl)
                n2212 = To Double Precision Float(number=w3784) -> (double precision float=w3783:dbl)
                n2213 = To Double Precision Float(number=w3793) -> (double precision float=w3792:dbl)
                n2214 = Multiply(x=w3799, y=w3777) -> (x*y=w3798:dbl)
                n2215 = To Double Precision Float(number=w3770) -> (double precision float=w3776:dbl)
                n2216 = Build Array(w3776, w3775, w3775, w3775, w3775) -> (w3773:dbl[])
                n2217 = local read "N sets should be saved"() -> (w3779:dbl)
                n2218 = Build Array(w3792, w3787, w3785, w3783, w3781) -> (w3789:dbl[])
                n2219 = Build Array(w3772, w3777, w3798, w3797, w3796, 2.0 ("t")) -> (w3791:dbl[])
                n2220 = Round Toward +Infinity(x=w3779) -> (ceil(x): smallest int >= x=w3780:dbl)
                n2221 = Build Array (concatenate)(w3791, w3790, w3773, w3789) -> (w3788:dbl[])
                n2222 = To Unsigned Long Integer(number=w3780) -> (unsigned 32bit integer=w3778:u32)
              }
              frame 8 {
                w3808 = 0.0 ("f")
                # "MCL raster scan"
                n2223 = local read "Number of scans (MCL)"() -> (w3803:u64)
                n2224 = local read "Scan lines (y)"() -> (w3802:u64)
                n2225 = local read "2D or 1D Scan"() -> (w3805:bool)
                n2226 = local read "Scan Range (V)\n(of steps)"() -> (w3824:dbl)
                n2227 = local read "Fast Scan Dir"() -> (w3831:bool)
                n2228 = local read "Cycles/step (MCL)"() -> (w3821:u64)
                n2229 = local read "Scan steps (MCL)"() -> (w3823:u64)
                n2230 = Select(t=w3802, s=w3805, f=w3803) -> (s? t:f=w3804:u64)
                n2231 = Boolean To (0,1)(Boolean=w3805) -> (0, 1=w3807:i16)
                n2232 = local read "Save ave N"() -> (w3836:dbl)
                n2233 = local read "Initial X"() -> (w3810:dbl)
                n2234 = local read "Initial Y"() -> (w3809:dbl)
                n2235 = To Double Precision Float(number=w3807) -> (double precision float=w3806:dbl)
                n2236 = Boolean To (0,1)(Boolean=w3831) -> (0, 1=w3830:i16)
                n2237 = To Double Precision Float(number=w3804) -> (double precision float=w3819:dbl)
                n2238 = To Double Precision Float(number=w3823) -> (double precision float=w3822:dbl)
                n2239 = To Double Precision Float(number=w3821) -> (double precision float=w3820:dbl)
                n2240 = To Double Precision Float(number=w3830) -> (double precision float=w3829:dbl)
                n2241 = Multiply(x=w3836, y=w3815) -> (x*y=w3835:dbl)
                n2242 = To Double Precision Float(number=w3800) -> (double precision float=w3814:dbl)
                n2243 = local read "N sets should be saved (MCL)"() -> (w3817:dbl)
                n2244 = Build Array(w3814, w3806, w3808, w3808, w3808) -> (w3812:dbl[])
                n2245 = Build Array(w3829, w3824, w3822, w3820, w3819, w3810, w3809) -> (w3826:dbl[])
                n2246 = Build Array(w3811, w3815, w3835, w3834, w3833, 3.0 ("t")) -> (w3828:dbl[])
                n2247 = Round Toward +Infinity(x=w3817) -> (ceil(x): smallest int >= x=w3818:dbl)
                n2248 = Build Array (concatenate)(w3828, w3827, w3812, w3826) -> (w3825:dbl[])
                n2249 = To Unsigned Long Integer(number=w3818) -> (unsigned 32bit integer=w3816:u32)
              }
            }
            n2250 = local read "Index"() -> (w3675:dbl)
            n2251 = call "Create new save file.vi"("Insert"="", "Ext"=".dat", "Index In"=w3675) -> ("Path Out"=w3634:path, "Index Out"=w3647:dbl)
            n2252 = local write "Save file name"(w3634) -> ()
            n2253 = local write "Index"(w3647) -> ()
            n2254 = local write "Save index"(w3647) -> ()
            n2255 = Array Size(array=w3658) -> (size(s)=w3659:i32)
            n2256 = Open/Create/Replace File(file path (use dialog)=w3634, operation (0:open)=T24."create", access (0:read/write)=enum16{"read/write", "read-only", "write-only"}."write-only") -> (refnum out=w3672:refnum<file>)  [unwired: 1 in, 4 out]
            n2257 = local write "Saving..."(TRUE ("Saving...")) -> ()
            n2258 = To Double Precision Float(number=w3659) -> (double precision float=w3657:dbl)
            n2259 = String Length(string="Comment (data description)") -> (length=w3655:i32)
            n2260 = To Double Precision Float(number=w3655) -> (double precision float=w3654:dbl)
            n2261 = Deny Access(7:w3672) -> (3:w3671:refnum<file>)  [unwired: 1 in, 2 out]
            n2262 = Build Array (concatenate)(w3657, w3658, w3654) -> (w3656:dbl[])
            n2263 = case "If fluorescence data to be saved" shown="True" w3645 {
              tunnel: w3634 -> [_ w3724]
              tunnel: [refnum<k0> refnum w3704] -> w3646
              frame False {
              }
              frame True {
                w3703 = 0.0
                n2264 = local read "APD Integration Time (s)"() -> (w3709:dbl)
                n2265 = local read "N APD Samp/step"() -> (w3702:dbl)
                n2266 = Path To String(path=w3724) -> (string=w3723:string)
                n2267 = String Length(string=w3723) -> (length=w3722:i32)
                n2268 = Subtract(x=w3722, y=4) -> (x-y=w3720:i32)
                n2269 = String Subset(string=w3723, length (rest)=w3720) -> (substring=w3719:string)  [unwired: 1 out]
                n2270 = Build Array(w3709, w3702, w3703, w3703, w3703, w3703, w3703, w3703) -> (w3706:dbl[])
                n2271 = Concatenate Strings(w3719, "_fl.dat" ("string")) -> (w3717:string)
                n2272 = Array Size(array=w3706) -> (size(s)=w3708:i32)
                n2273 = String To Path(string=w3717) -> (path=w3713:path)
                n2274 = Open/Create/Replace File(file path (use dialog)=w3713, operation (0:open)=T24."create", access (0:read/write)=enum16{"read/write", "read-only", "write-only"}."write-only") -> (refnum out=w3714:refnum<file>)  [unwired: 1 in, 4 out]
                n2275 = Deny Access(7:w3714) -> (3:w3710:refnum<file>)  [unwired: 1 in, 2 out]
                n2276 = To Double Precision Float(number=w3708) -> (double precision float=w3707:dbl)
                n2277 = Build Array (concatenate)(w3707, w3706) -> (w3705:dbl[])
                n2278 = Write to Binary File(file (use dialog)=w3710, data=w3705, 5:FALSE ("prepend array or string size? (T)"), 9:T30."big-endian, network order" ("byte order (0:big-endian, network order)")) -> (refnum out=w3704:refnum<file>)  [unwired: 1 in, 3 out]
              }
            }
            n2279 = case shown="True" w3632 {
              tunnel: w3634 -> [_ w3686]
              tunnel: [refnum<k0> refnum w3685] -> w3633
              frame False {
              }
              frame True {
                w3681 = 0.0 ("element")
                n2280 = Path To String(path=w3686) -> (string=w3700:string)
                n2281 = Build Array(w3681, w3681, w3681, w3681, w3681, w3681, w3681, w3681) -> (w3682:dbl[])
                n2282 = String Length(string=w3700) -> (length=w3699:i32)
                n2283 = Subtract(x=w3699, y=4) -> (x-y=w3697:i32)
                n2284 = Array Size(array=w3682) -> (size(s)=w3684:i32)
                n2285 = String Subset(string=w3700, length (rest)=w3697) -> (substring=w3696:string)  [unwired: 1 out]
                n2286 = To Double Precision Float(number=w3684) -> (double precision float=w3683:dbl)
                n2287 = Concatenate Strings(w3696, "_pos.dat" ("string")) -> (w3694:string)
                n2288 = Build Array (concatenate)(w3683, w3682) -> (w3680:dbl[])
                n2289 = String To Path(string=w3694) -> (path=w3690:path)
                n2290 = Open/Create/Replace File(file path (use dialog)=w3690, operation (0:open)=T24."create", access (0:read/write)=enum16{"read/write", "read-only", "write-only"}."write-only") -> (refnum out=w3691:refnum<file>)  [unwired: 1 in, 4 out]
                n2291 = Deny Access(7:w3691) -> (3:w3687:refnum<file>)  [unwired: 1 in, 2 out]
                n2292 = Write to Binary File(file (use dialog)=w3687, data=w3680, 5:FALSE ("prepend array or string size? (T)"), 9:T30."big-endian, network order" ("byte order (0:big-endian, network order)")) -> (refnum out=w3685:refnum<file>)  [unwired: 1 in, 3 out]
              }
            }
            n2293 = Write to Binary File(file (use dialog)=w3671, data=w3656, 5:w3652, 9:w3650) -> (refnum out=w3653:refnum<file>)  [unwired: 1 in, 3 out]
            n2294 = Write to Binary File(file (use dialog)=w3653, data="Comment (data description)", 5:w3652, 9:w3650) -> (refnum out=w3649:refnum<file>)  [unwired: 1 in, 3 out]
          }
        }
        n2295 = feedback-in #19(w3592) -> ()
        n2296 = feedback-in #20(w3619) -> ()
        n2297 = feedback-in #21(w3591) -> ()
        n2298 = feedback-in #22(w3602) -> ()
        n2299 = feedback-in #23(w3605) -> ()
        n2300 = feedback-in #24(w3618) -> ()
        n2301 = feedback-in #25(w3608) -> ()
      }
      frame #1 {
        n2302 = local read "Saving..."() -> (w3849:bool)
        n2303 = case shown="True" w3849 {
          tunnel: w3853 -> [_ w3863]
          tunnel: w3852 -> [_ w3877]
          tunnel: w3851 -> [_ w3873]
          tunnel: w3850 -> [_ w3872]
          tunnel: w3848 -> [_ w3871]
          tunnel: w3847 -> [_ w3866]
          tunnel: w3846 -> [_ w3865]
          tunnel: w3845 -> [_ w3864]
          tunnel: w3844 -> [_ w3862]
          tunnel: w3843 -> [_ w3860]
          tunnel: w3842 -> [_ w3859]
          tunnel: w3841 -> [_ w3858]
          tunnel: w3840 -> [_ w3857]
          tunnel: w3839 -> [_ w3856]
          tunnel: w3838 -> [_ w3855]
          tunnel: w3837 -> [_ w3854]
          frame False {
          }
          frame True {
            n2304 = Multiply(x=w3863, y=w3862) -> (x*y=→"Time (s)":dbl)
            n2305 = Less Or Equal?(x=w3863, y=w3871) -> (x <= y?=w3875:bool)
            n2306 = Or(x="Stop Saving", y="Abort save 2") -> (x .or. y?=w3867:bool)
            n2307 = Not(x=w3867) -> (.not. x?=w3876:bool)
            n2308 = And(x=w3875, y=w3876) -> (x .and. y?=w3874:bool)
            n2309 = case shown="True" w3874 {
              tunnel: w3877 -> [w3884 w3952]
              tunnel: [0.0 w3955] -> w3870
              tunnel: w3863 -> [_ w3953]
              tunnel: w3871 -> [_ w3954]
              tunnel: w3873 -> [_ w3949]
              tunnel: w3872 -> [_ _]
              tunnel: w3866 -> [w3882 w3942]
              tunnel: w3865 -> [w3881 w3943]
              tunnel: w3864 -> [_ w3941]
              tunnel: w3860 -> [_ w3940]
              tunnel: w3859 -> [_ w3894]
              tunnel: w3858 -> [_ w3933]
              tunnel: w3857 -> [_ w3911]
              tunnel: w3856 -> [w3879 w3892]
              tunnel: w3855 -> [w3880 w3891]
              tunnel: w3854 -> [_ w3888]
              frame False {
                w3878 = FALSE
                n2310 = Close File(refnum=w3884) -> ()  [unwired: 1 in, 2 out]
                n2311 = case shown="True" w3881 {
                  tunnel: w3882 -> [_ w3886]
                  frame False {
                  }
                  frame True {
                    n2312 = Close File(refnum=w3886) -> ()  [unwired: 1 in, 2 out]
                  }
                }
                n2313 = case shown="True" w3879 {
                  tunnel: w3880 -> [_ w3885]
                  frame False {
                  }
                  frame True {
                    n2314 = Close File(refnum=w3885) -> ()  [unwired: 1 in, 2 out]
                  }
                }
                n2315 = local write "Calibrating Trap..."(w3878) -> ()
                n2316 = call <vilib>:"Beep.vi"() -> ()  [unwired: 3 in, 9 out]
                n2317 = local write "Stop Saving"(w3878) -> ()
                n2318 = property on="Raster Scanning..." class="Bool (strict)"("Val(Sgnl)"=w3878) -> ()  [unwired: 2 in, 2 out]
                "Saving..." <- w3878
              }
              frame True {
                n2319 = local read "Calibrating Trap..."() -> (w3944:bool)
                n2320 = case "Write fl. data" shown="True" w3943 {
                  tunnel: w3942 -> [_ w3978]
                  tunnel: w3941 -> [_ w3977]
                  frame False {
                  }
                  frame True {
                    n2321 = Write to Binary File(file (use dialog)=w3978, data=w3977, 5:FALSE ("prepend array or string size? (T)"), 9:T30."big-endian, network order" ("byte order (0:big-endian, network order)")) -> ()  [unwired: 1 in, 4 out]
                  }
                }
                n2322 = Greater?(x="Save ave N", y=1.0) -> (0:w3947:bool)
                n2323 = Not(x=w3944) -> (.not. x?=w3946:bool)
                n2324 = And(x=w3946, y=w3947) -> (x .and. y?=w3889:bool)
                n2325 = case shown="True" w3889 {
